vi "TLB Native Dynamic Events ver 0.08d.vi"() -> ()   [LabVIEW 2018]
uses:
  Labview Training Phase 2/Enum Controls/States for Action Engine.ctl
  Type def/TLB event states.ctl
  Type def/TLB MHL States.ctl
  <vilib>/Studica/Studica Toolkit/Background/I2C Channel.ctl
  <vilib>/myRIO/Common/Instrument Driver Framework/myRIO v1.0/AI/typedefs/AI Channels Enum.ctl
  <vilib>/myRIO/Common/Instrument Driver Framework/myRIO v1.0/AI/typedefs/AI Channels List.ctl
  Type def/Type def.ctl
  <vilib>/Studica/Studica Blackhawk/Blackhawk.lvlib
  <vilib>/Studica/Studica Toolkit/Background/Mxp Selection.ctl
  <vilib>/Studica/Studica Toolkit/Background/DIO Channel.ctl
  <vilib>/NI_Real-Time Target Support.lvlib
  <vilib>/ptbypt/NI_PtbyPt.lvlib
  <vilib>/addons/control/pid/NI_PID_pid.lvlib
  Underlying VI's/Webcam FGV Low level ver/State control.ctl
  <vilib>/userdefined/High Color/IMAQdx.ctl
  <vilib>/Studica/Studica Toolkit/NavX/NavX.lvlib
  <vilib>/addons/control/pid/pid.llb/PID (DBL).vi
  Underlying VI's/Movement control (archived)/Motor Control/States for motor control.ctl
panel:
  out "Displacement":T1
  out "Yaw":dbl
  out "Speed and distance cluster":T2
  out "Output":dbl
  in  "SENSOR":bool
  out "Decision":i8
  out "Manual Zero Yaw":bool
  in  "error in (no error)":errorcluster
  in  "RED LED State":enum16{"OFF", "ON", "BLINK"}(ring)
  in  "GREEN LED State":enum16{"OFF", "ON", "BLINK"}(ring)
  in  "Red LED":bool
  in  "Green LED":bool
  out "Input state":i8
  out "Waveform Chart 2":dbl(graph)
  out "Waveform Chart":dbl(graph)
  in  "STOP":bool
  out "DIO 0":bool
  out "DIO 1":bool
  out "Limit Switch Array":bool[](array[boolean])
  out "error out":errorcluster
  out "L/R average":fxp<+,64,64>
  out "Right Ultrasonic":fxp<+,64,16>
  out "Left Ultrasonic":fxp<+,64,16>
  out "Right IR Sensor":dbl
  out "Left IR Sensor":dbl
  out "Object detection count":T3
  out "Camera error":errorcluster
  in  "Servo Angle":u8(slide) scale=0.0..180.0
  in  "On/Off":bool
  out "Error":errorcluster
  out "element":T4
  out "Action Queue Items":i32
  out "State Logic Queue Items":i32
  out "Action Queues items":string[](array[string])=["Hardware reset", "Software reset", ""]
  out "State logic":T5=enum."Task 2"
  out "Action State":string
  # "TLB FRAMEWORK STATUS"
  # "Camera Status Loop"
  # "Test Programme written by Calvin Loke    Dated: 28 Aug 2019\nTest Programme revised by Dr Alex See   Dated 30 Aug 2019\n\nProgramme version:   TLB Native Dynamic Events ver 0.04b.vi"
  # "Problems now:\nYaw does not work when code is in last state mode\nSlow acceleration due to loop rate?"
  # "Motor Control Loop"
  # "NAVX Control Loop"
  # "Blackhawk status"
  # "Sensor data"
  # "System Health Status Update"
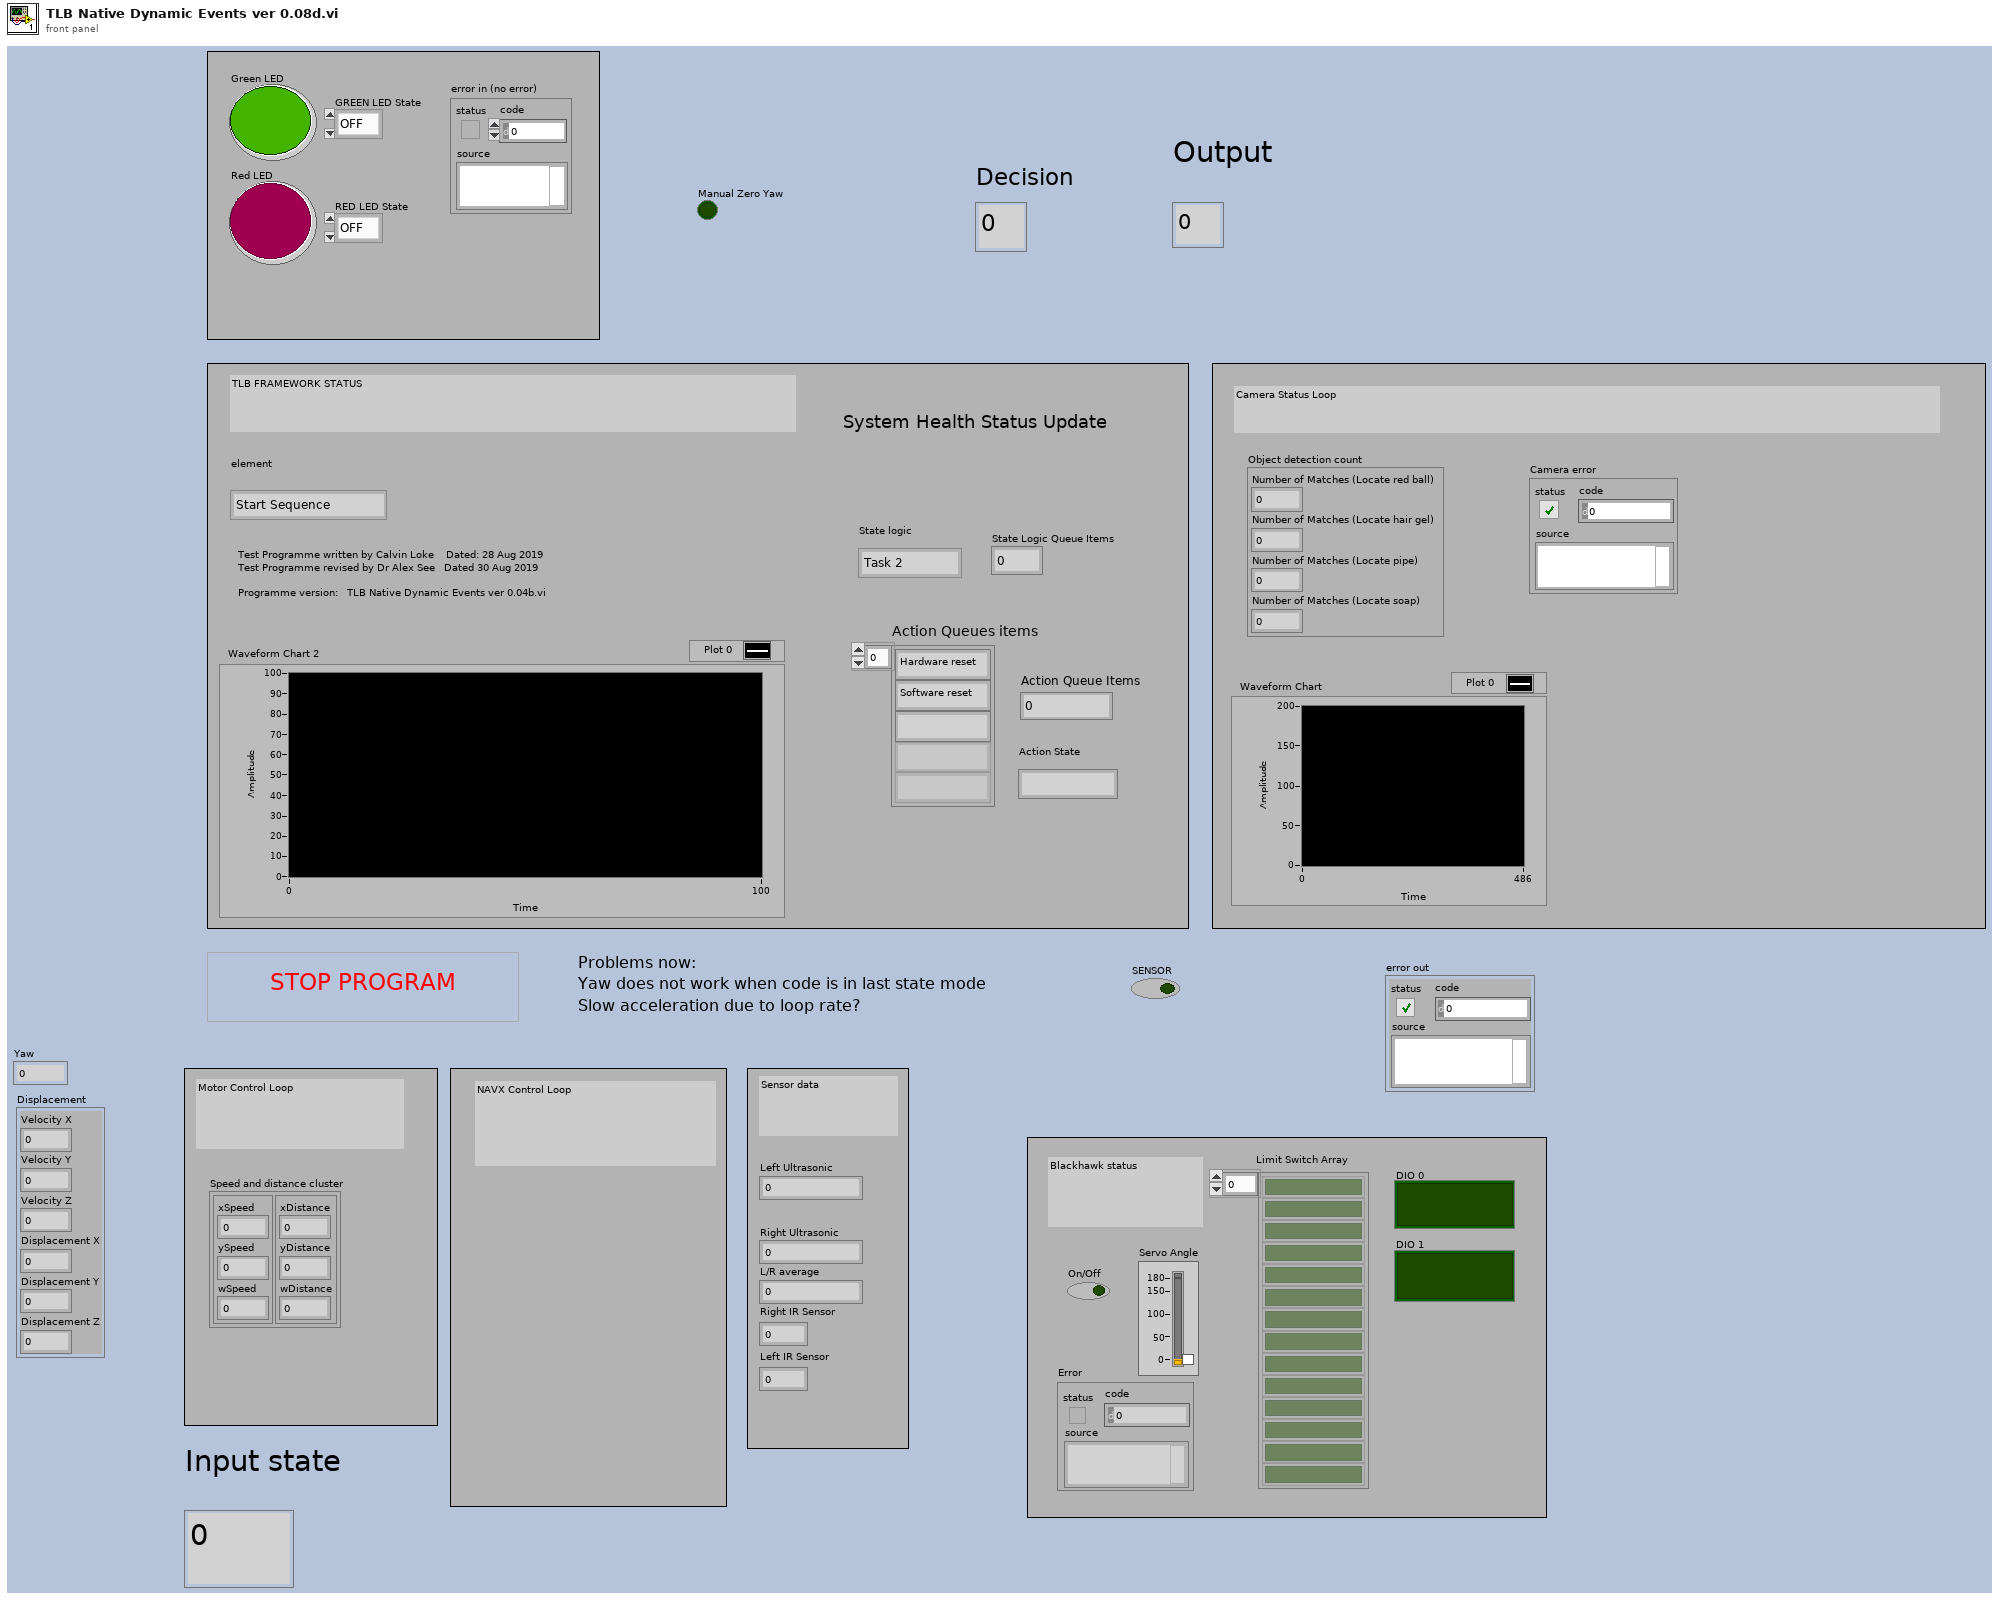
[diagram p1: front panel]
types:
  T1 = cluster{"Velocity X":dbl, "Velocity Y":dbl, "Velocity Z":dbl, "Displacement X":dbl, "Displacement Y":dbl, "Displacement Z":dbl}
  T2 = cluster{cluster{"xSpeed":dbl, "ySpeed":dbl, "wSpeed":dbl}, cluster{"xDistance":dbl, "yDistance":dbl, "wDistance":dbl}}
  T3 = cluster{"Number of Matches (Locate red ball)":i32, "Number of Matches (Locate hair gel)":i32, "Number of Matches (Locate pipe)":i32, "Number of Matches (Locate soap)":i32}
  T4 = typedef "TLB event states.ctl" = enum16{"Start Sequence", "Exit", "Start Task 1", "Start Task 2", "Start Task 3", "Start Task 4", "Camera vision", "Wall follow mode", "Idle", "Start Drive Straight"}
  T5 = typedef "TLB MHL States.ctl" = enum16{"None", "Startup", "Idle", "Processing", "Shutdown", "Reset", "Task 1", "Task 2", "Task 3", "Task 4", "Task 4a", "Task 4b", "Task 4c", "Task 4d", "Task 4e", "Task 4f", "Task 4g", "Task 4h", "Acquire image", "Wall follow mode", "Autodrive", "Autodrive a"}
  T6 = typedef "States for motor control.ctl" = enum16{"LAST STATE", "STOP", "FORWARD", "BACKWARD", "LEFT", "RIGHT", "RCW", "ACW", "INIT", "RESET ENCODERS"}
  T7 = typedef "States for Action Engine.ctl" = enum16{"Initialize", "Write", "Read"}
  T8 = typedef "DIO Channel.ctl" = enum16{"Not Connected", "A/DIO1", "A/DIO2", "A/DIO3", "A/DIO4", "A/DIO5", "A/DIO6", "A/DIO7", "A/DIO13", "B/DIO1", "B/DIO2", "B/DIO3", "B/DIO4", "B/DIO5", "B/DIO6", "B/DIO7", "B/DIO13", "C/DIO0", "C/DIO1", "C/DIO2", "C/DIO3", "C/DIO4", "C/DIO5", "C/DIO6", "C/DIO7"}
  T9 = typedef "Type def.ctl" = cluster{"Front Ultrasonic Obstruct":bool, "Left Ultrasonic Obstruct":bool, "Right Ultrasonic Obstruct ":bool}
  T10 = typedef "I2C Channel.ctl" = enum16{"Not Connected", "A", "B"}
  T11 = enum16{"LAST STATE", "STOP", "FORWARD", "BACKWARD", "LEFT", "RIGHT", "RCW", "ACW", "INIT", "RESET ENCODERS"}
  T12 = cluster{"proportional gain (Kc)":dbl, "integral time (Ti, min)":dbl, "derivative time (Td, min)":dbl}
  T13 = typedef "State control.ctl" = enum16{"Initialise", "Start camera", "Continuous Acquisition ", "Stop camera", "Dispose all"}
  T14 = typedef "IMAQdx.ctl" = refnum<k21>
  T15 = typedef "Mxp Selection.ctl" = enum16{"MXP A", "MXP B"}
  T16 = typedef "AI Channels List.ctl" = T17[]
  T17 = typedef "AI Channels Enum.ctl" = enum16{"Not Connected", "AudioIn/Left", "AudioIn/Right", "C/AI0", "C/AI1", "A/AI0", "A/AI1", "A/AI2", "A/AI3", "A/AI4", "A/AI5", "A/AI6", "A/AI7", "B/AI0", "B/AI1", "B/AI2", "B/AI3", "B/AI4", "B/AI5", "B/AI6", "B/AI7", "AI/AI0", "AI/AI1", "AI/AI2", "AI/AI3", "A/AI0 (DIFF)", "A/AI1 (DIFF)", "A/AI2 (DIFF)", "A/AI3 (DIFF)", "B/AI0 (DIFF)", "B/AI1 (DIFF)", "B/AI2 (DIFF)", "B/AI3 (DIFF)"}
  T18 = cluster{"DIO Channel":T8, "FPGA VI Reference Out":refnum<k20>}
  T19 = typedef "Analog Scaling Constants List.ctl" = T20[]
  T20 = typedef "Analog Scaling Constants.ctl" = cluster{"LSB Weight (Volts)":dbl, "Offset (Volts)":dbl, "Signed?":bool}
  T21 = cluster{"Scale Constants Array":T19, "FPGA Reference Out":refnum<k20>, "AI Channel":T16}
  T22 = cluster{"I2C Channel":T10, "FPGA VI Reference Out":refnum<k20>}
  T23 = typedef "NI_Real-Time Target Support.lvlib/RT CPU Load.ctl" = cluster{"Total (%)":dbl, "Time Critical (%)":dbl, "Timed Structures (%)":dbl, "High (%)":dbl, "Above Normal (%)":dbl, "Normal (%)":dbl, "Background (%)":dbl, "Idle (%)":dbl, "ISR (%)":dbl}
  T24 = cluster{"CPU loads[0]":T23, "CPU loads[1]":T23, "CPU loads[2]":T23, "CPU loads[3]":T23, "CPU loads[4]":T23, "CPU loads[5]":T23, "CPU loads[6]":T23, "CPU loads[7]":T23, "CPU loads[8]":T23}
  T25 = cluster{"I2C Ref Out":cluster{"I2C Channel":T10, "FPGA VI Reference Out":refnum<k20>}, "Connected":bool, "Slave Address (7-bit)":u8, "Registry":u8[]}
  T26 = typedef "IMAQ Image.ctl" = refnum<image>
  T27 = cluster{"Yaw":dbl, "Roll":dbl, "Pitch":dbl, "Heading":dbl, "Fused Heading":dbl}
  T28 = cluster{"xDistance":dbl, "yDistance":dbl, "wDistance":dbl}
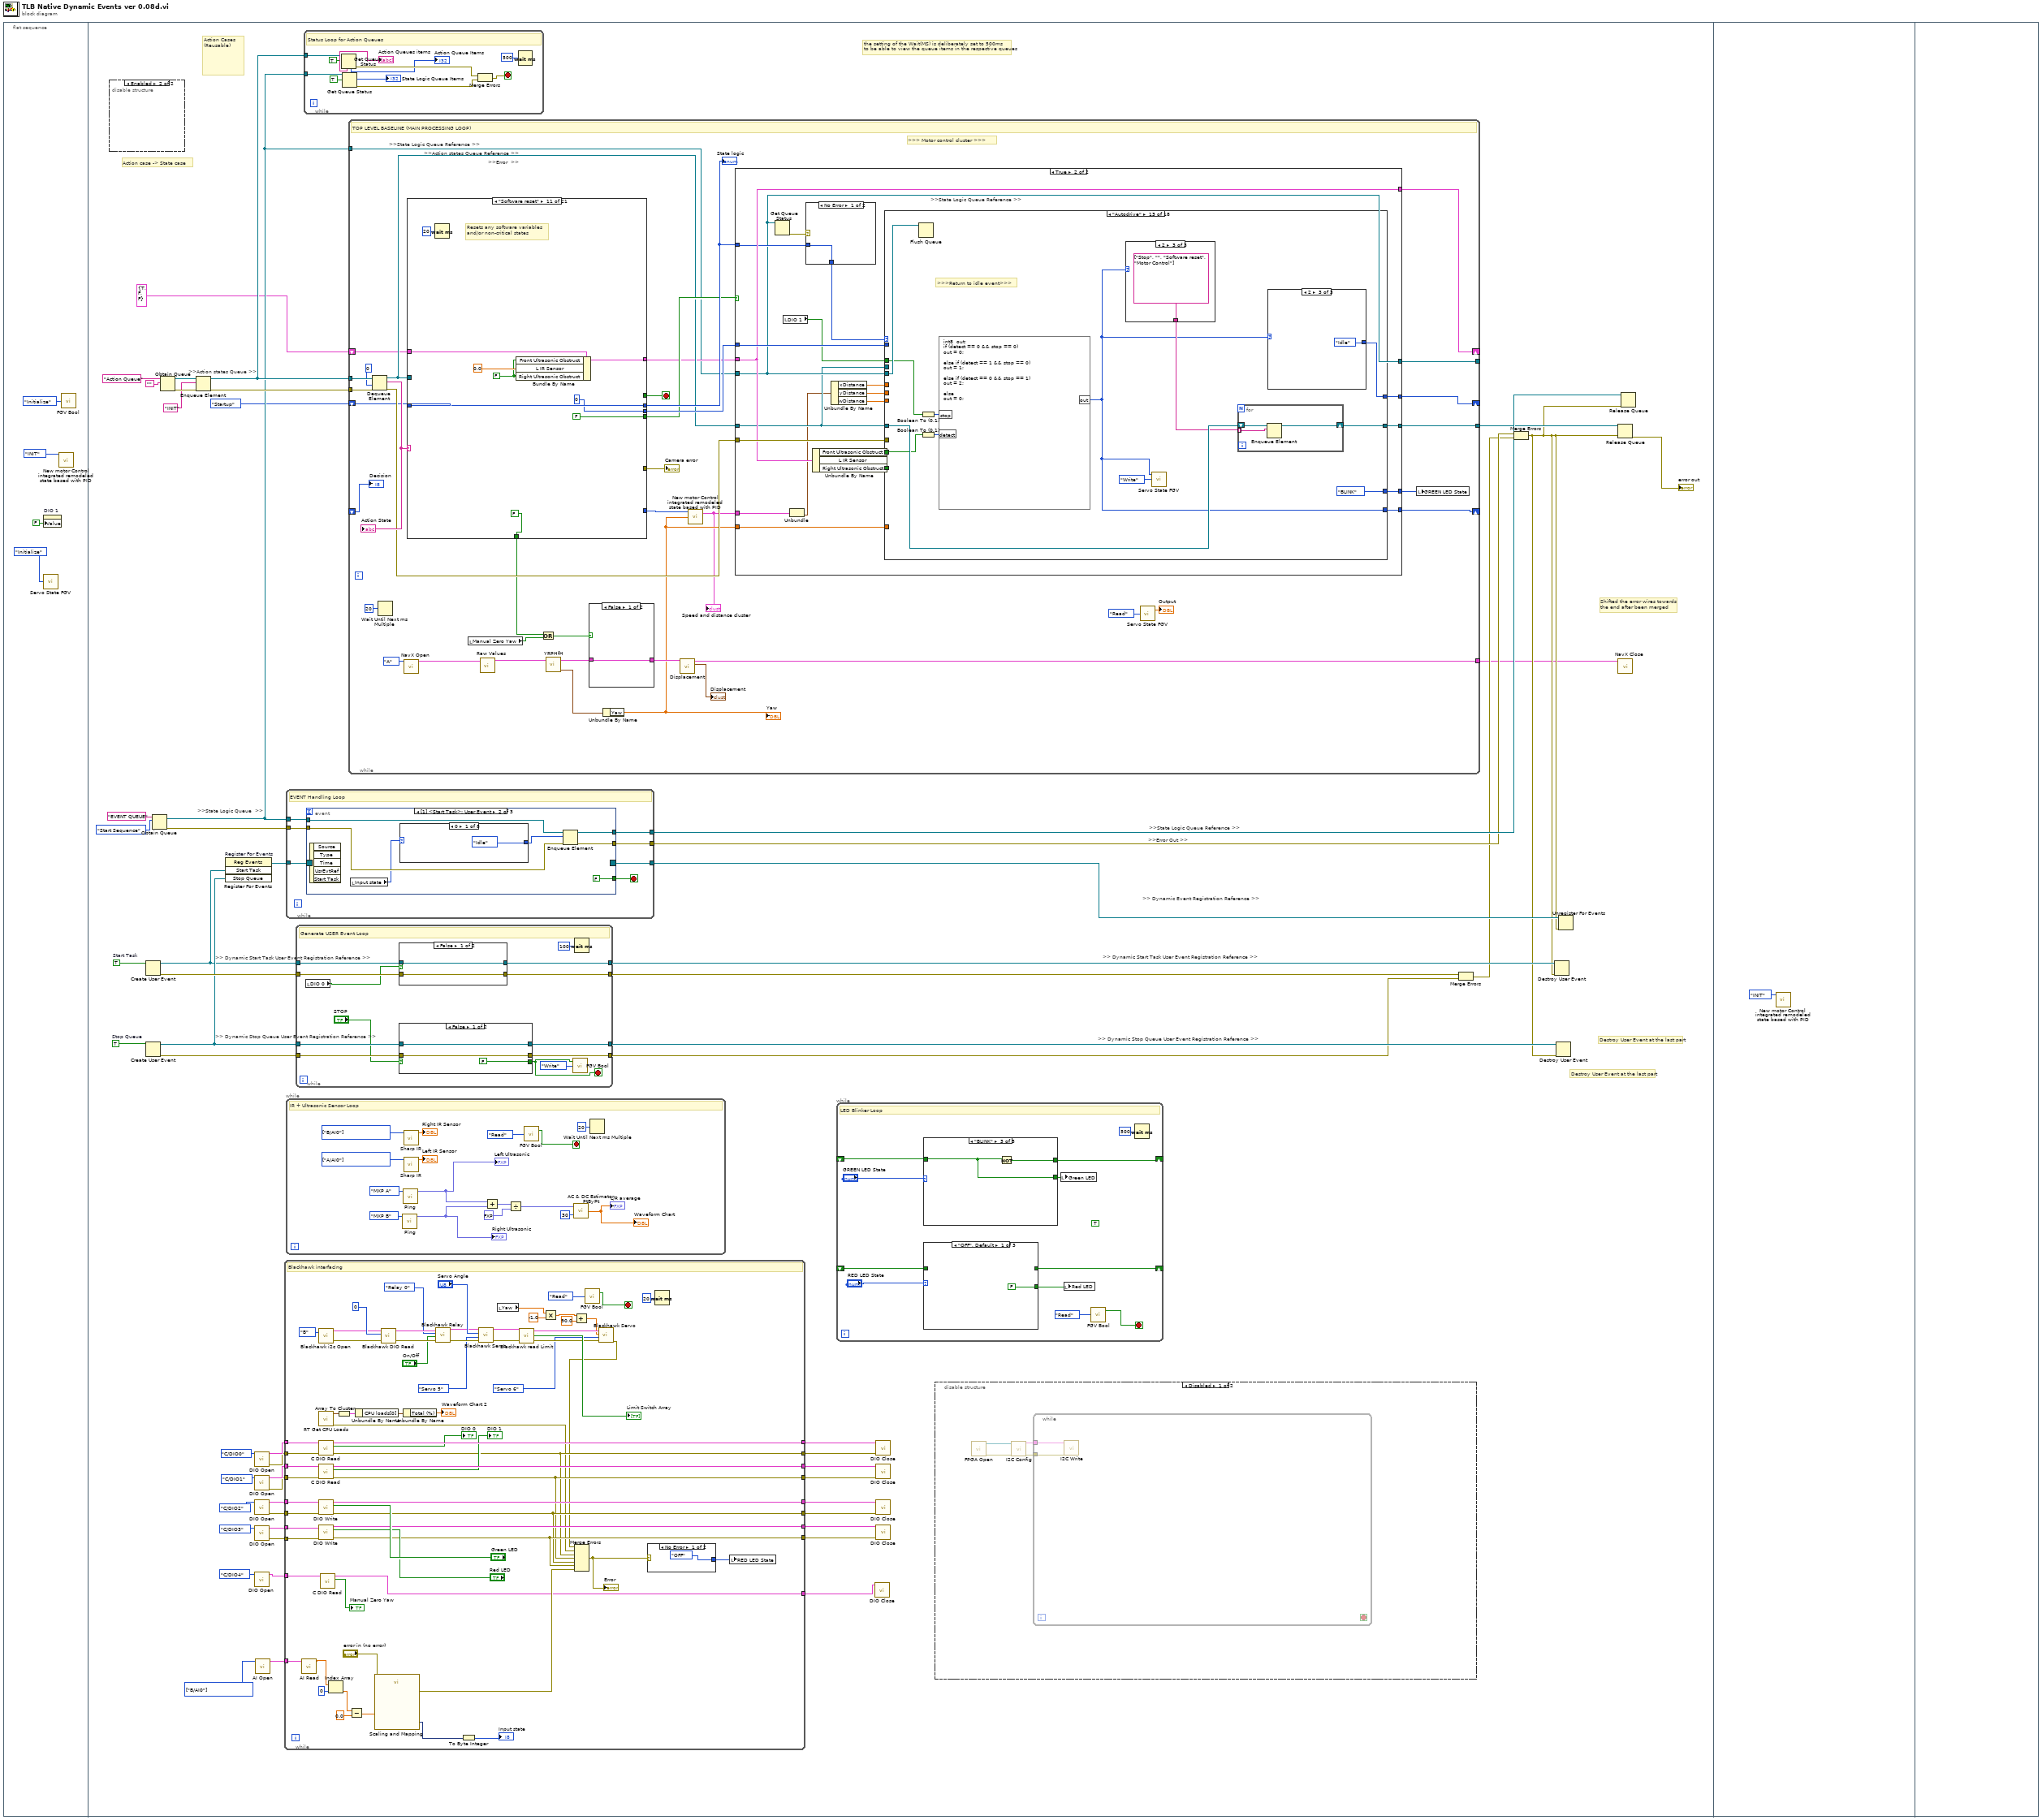
[diagram p0: block diagram]
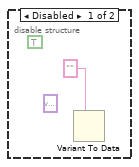
[diagram p3: hidden frame]
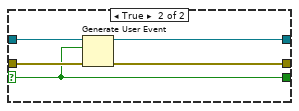
[diagram p4: hidden frame]
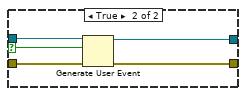
[diagram p5: hidden frame]
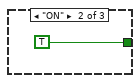
[diagram p6: hidden frame]
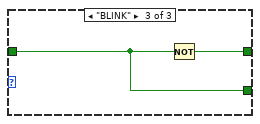
[diagram p7: hidden frame]
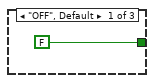
[diagram p8: hidden frame]
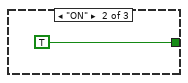
[diagram p9: hidden frame]
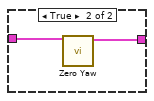
[diagram p10: hidden frame]
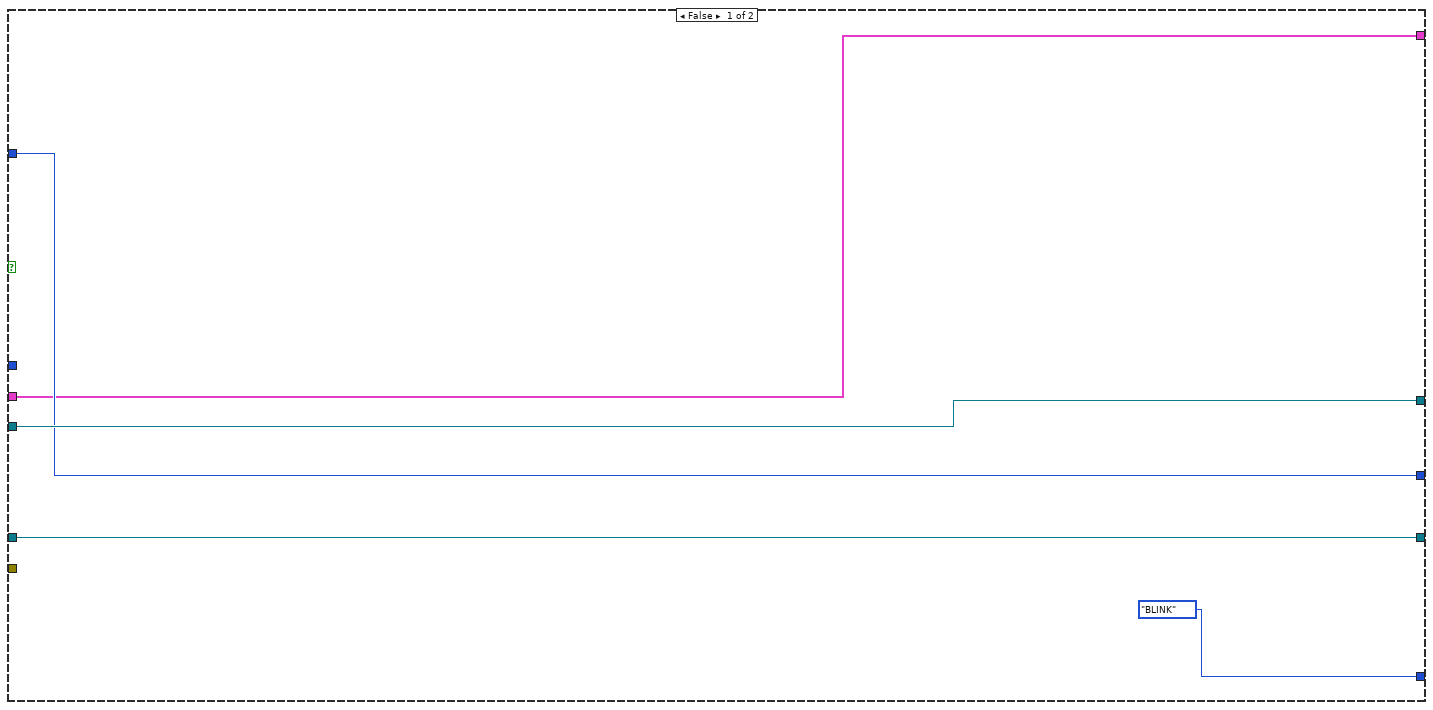
[diagram p11: hidden frame]
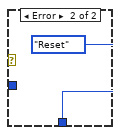
[diagram p12: hidden frame]
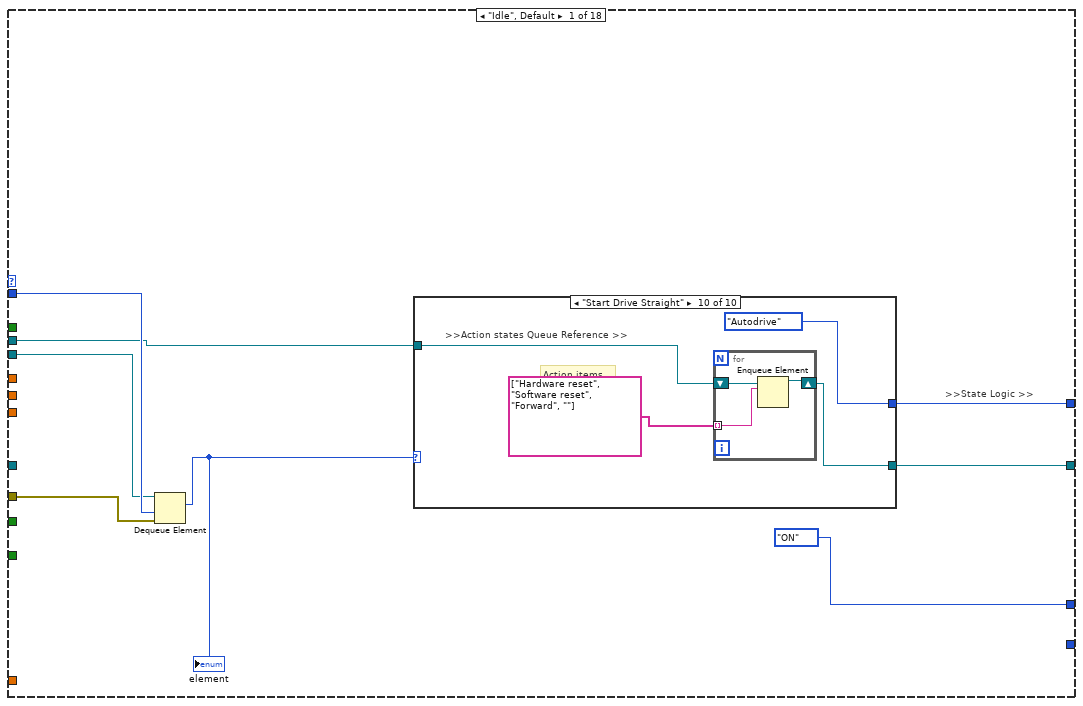
[diagram p13: hidden frame]
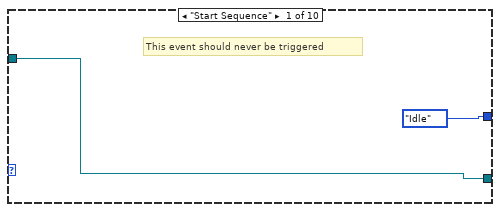
[diagram p14: hidden frame]
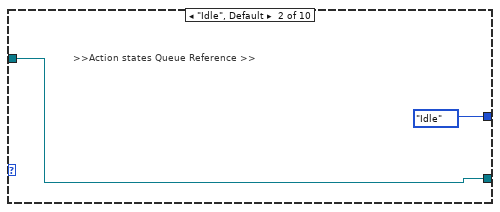
[diagram p15: hidden frame]
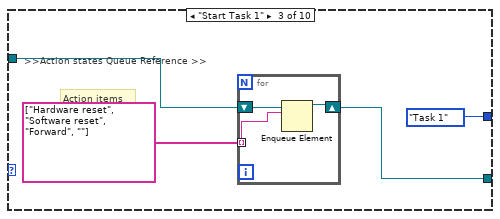
[diagram p16: hidden frame]
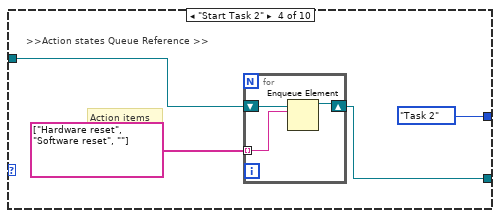
[diagram p17: hidden frame]
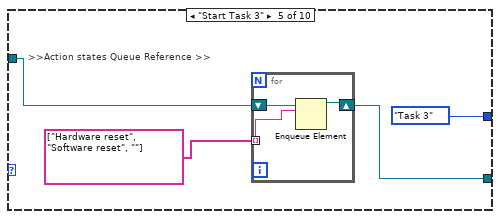
[diagram p18: hidden frame]
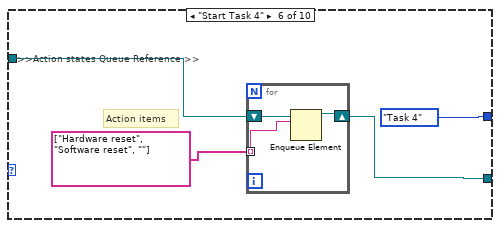
[diagram p19: hidden frame]
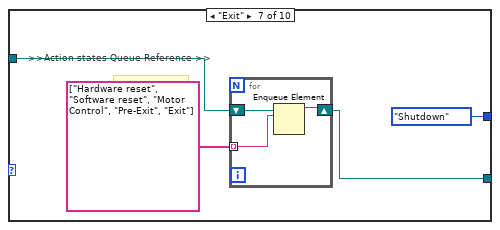
[diagram p20: hidden frame]
diagram:
  n1 = flat-sequence {
    frame #0 {
      n2 = call "Servo State FGV.vi"("Init/Read/Write State"=States_for_Action_Engine."Initialize") -> ()  [unwired: 2 in, 2 out]
      n3 = property on="DIO 1" class="Bool (strict)"("Value"=FALSE ("DIO 1")) -> ()  [unwired: 2 in, 2 out]
      n4 = call "New motor Control integrated remodeled state based with PID.vi"("States"=States_for_motor_control."INIT") -> ()  [unwired: 2 in, 2 out]
      n5 = call "FGV Bool.vi"("Init/Read/Write State"=States_for_Action_Engine."Initialize") -> ()  [unwired: 2 in, 2 out]
    }
    frame #1 {
      w14 = T16 [enum."B/AI0"] items=["Not Connected", "AudioIn/Left", "AudioIn/Right", "C/AI0", "C/AI1", "A/AI0", "A/AI1", "A/AI2", "A/AI3", "A/AI4", "A/AI5", "A/AI6", "A/AI7", "B/AI0", "B/AI1", "B/AI2", "B/AI3", "B/AI4", "B/AI5", "B/AI6", "B/AI7", "AI/AI0", "AI/AI1", "AI/AI2", "AI/AI3", "A/AI0 (DIFF)", "A/AI1 (DIFF)", "A/AI2 (DIFF)", "A/AI3 (DIFF)", "B/AI0 (DIFF)", "B/AI1 (DIFF)", "B/AI2 (DIFF)", "B/AI3 (DIFF)"] ("AI Channel")
      w61 = TRUE  # Stop Queue
      w60 = TRUE  # Start Task
      # "Action case -> State case"
      # "the setting of the Wait(MS) is deliberately set to 500ms\nto be able to view the queue items in the respective queues"
      # "Action Cases\n(Reusable)"
      # ">>Error Out >>"
      # ">> Dynamic Stop Queue User Event Registration Reference >>"
      # ">> Dynamic Start Task User Event Registration Reference >>"
      # ">> Dynamic Stop Queue User Event Registration Reference >>"
      # ">> Dynamic Start Task User Event Registration Reference >>"
      # ">> Dynamic Event Registration Reference >>"
      # ">>Action states Queue >>"
      # ">>State Logic Queue  >>"
      # ">>State Logic Queue Reference >>"
      # "Destroy User Event at the last part"
      # "Destroy User Event at the last part"
      # "Shifted the error wires towards\nthe end after been merged"
      n6 = disable-structure shown="Enabled" {
        frame Disabled {
          (unwired) variant
          (unwired) TRUE
          n7 = Variant To Data(type="") -> ()  [unwired: 2 in, 2 out]
        }
        frame Enabled {
        }
      }
      n8 = Create User Event(user event datatype=w60) -> (user event=w52:refnum<user-event>, error out=w57:errorcluster)  [unwired: 1 in]
      n9 = Create User Event(user event datatype=w61) -> (user event=w53:refnum<user-event>, error out=w56:errorcluster)  [unwired: 1 in]
      n10 = Obtain Queue(name (unnamed)="EVENT QUEUE", element data type=TLB_event_states."Start Sequence" ("Enum")) -> (queue out=w37:refnum<queue>, error out=w43:errorcluster)  [unwired: 3 in, 1 out]
      n11 = Obtain Queue(name (unnamed)="Action Queue", element data type="") -> (queue out=w46:refnum<queue>, error out=w42:errorcluster)  [unwired: 3 in, 1 out]
      n12 = Enqueue Element(queue=w46, element="INIT", error in (no error)=w42) -> (queue out=w38:refnum<queue>, error out=w41:errorcluster)  [unwired: 1 in, 1 out]
      n13 = register-events "Register For Events"(w52, w53) -> (reference out=w51:refnum<event-registration>)  [unwired: 2 in, 1 out]
      n14 = call <vilib>:"DIO Open.vi"("DIO Channel"=DIO_Channel."C/DIO4") -> ("DIO Info Out"=w8:T18)  [unwired: 9 in, 1 out]
      n15 = call <vilib>:"DIO Open.vi"("DIO Channel"=DIO_Channel."C/DIO0") -> ("error out"=w24:errorcluster, "DIO Info Out"=w30:T18)  [unwired: 9 in]
      n16 = call <vilib>:"DIO Open.vi"("DIO Channel"=DIO_Channel."C/DIO1") -> ("error out"=w22:errorcluster, "DIO Info Out"=w26:T18)  [unwired: 9 in]
      n17 = call <vilib>:"DIO Open.vi"("DIO Channel"=DIO_Channel."C/DIO2") -> ("error out"=w12:errorcluster, "DIO Info Out"=w18:T18)  [unwired: 9 in]
      n18 = call <vilib>:"DIO Open.vi"("DIO Channel"=DIO_Channel."C/DIO3") -> ("error out"=w10:errorcluster, "DIO Info Out"=w17:T18)  [unwired: 9 in]
      n19 = call <vilib>:"AI Open.vi"("AI Channel"=w14) -> ("Analog Info"=w13:T21)  [unwired: 9 in, 1 out]
      n20 = while {
        tunnel: w30 -> [w743]
        tunnel: [w742] -> w29
        tunnel: w26 -> [w741]
        tunnel: [w740] -> w25
        tunnel: w24 -> [w739]
        tunnel: [w708] -> w23
        tunnel: w22 -> [w738]
        tunnel: [w709] -> w21
        tunnel: w18 -> [w732]
        tunnel: w17 -> [w731]
        tunnel: [w728] -> w16
        tunnel: [w727] -> w15
        tunnel: w13 -> [w726]
        tunnel: w12 -> [w719]
        tunnel: [w710] -> w11
        tunnel: w10 -> [w718]
        tunnel: [w711] -> w9
        tunnel: w8 -> [w699]
        tunnel: [w698] -> w6
        stop <- w756 stop-if-true
        # "Blackhawk interfacing"
        n21 = call <vilib>:"AI Read.vi"("Analog Info"=w726) -> ("Array"=w722:dbl[])  [unwired: 9 in, 1 out]
        n22 = call <vilib>:"Blackhawk i2c Open.vi"("I2C Channel"=I2C_Channel."B") -> ("I2C Ref Out"=w734:T22, "error out"=w733:errorcluster)  [unwired: 2 in]
        n23 = call <vilib>:"RT Get CPU Loads.vi"() -> ("error out"=w707:errorcluster, "CPU loads"=w713:T23[])  [unwired: 10 in]
        n24 = call <vilib>:"C DIO Read.vi"("error in (no error)"=w739, "DIO Info In in"=w743) -> ("error out"=w708:errorcluster, "IN"=→"DIO 0":bool, "DIO Info In out"=w742:T18)  [unwired: 7 in]
        n25 = call <vilib>:"C DIO Read.vi"("error in (no error)"=w738, "DIO Info In in"=w741) -> ("error out"=w709:errorcluster, "IN"=→"DIO 1":bool, "DIO Info In out"=w740:T18)  [unwired: 7 in]
        n26 = call <vilib>:"DIO Write.vi"("error in (no error)"=w719, "Input"="Green LED", "DIO Info In"=w732) -> ("error out"=w710:errorcluster, "DIO Info Out"=w728:T18)  [unwired: 7 in]
        n27 = call <vilib>:"DIO Write.vi"("error in (no error)"=w718, "Input"="Red LED", "DIO Info In"=w731) -> ("error out"=w711:errorcluster, "DIO Info Out"=w727:T18)  [unwired: 7 in]
        n28 = call <vilib>:"C DIO Read.vi"("DIO Info In in"=w699) -> ("IN"=→"Manual Zero Yaw":bool, "DIO Info In out"=w698:T18)  [unwired: 8 in, 1 out]
        n29 = Index Array(array=w722, index=0) -> (element=w724:dbl)
        n30 = Array To Cluster(array=w713) -> (cluster=w714:T24)
        n31 = Subtract(x=w724, y=0.0) -> (x-y=w725:dbl)
        n32 = Unbundle By Name(w714) -> ("CPU loads[0]"=w715:T23)
        n33 = call "Scaling and Mapping"("error in (no error)"="error in (no error)", "Signals"=w725) -> ("error out"=w712:errorcluster, "Scaled Signals"=w720:dynamicdata)  [unwired: 8 in]
        n34 = call <vilib>:"Blackhawk DIO Read.vi"("I2C Ref In"=w734, "PIN"=u8 0, "error in (no error)"=w733) -> ("I2C Ref Out"=w754:T22, "error out"=w755:errorcluster)  [unwired: 3 in, 1 out]
        n35 = Unbundle By Name(w715) -> ("Total (%)"=→"Waveform Chart 2":dbl)
        n36 = call <vilib>:"Blackhawk Relay.vi"("error in (no error)"=w755, "On/Off"="On/Off", "Relay"=enum8{"Relay 0", "Relay 1", "Relay 2"}."Relay 0", "I2C Ref In"=w754) -> ("error out"=w751:errorcluster, "I2C Ref Out"=w748:T22)  [unwired: 6 in]
        n37 = To Byte Integer(number=w720) -> (8bit integer=→"Input state":i8)
        n38 = call <vilib>:"Blackhawk Servo.vi"("error in (no error)"=w751, "Servo Select"=enum16{"Servo 5", "Servo 6"}."Servo 5", "Servo Angle"="Servo Angle", "I2C Ref In"=w748) -> ("error out"=w746:errorcluster, "I2C Ref Out"=w745:T22)  [unwired: 6 in]
        n39 = local read "Yaw"() -> (w692:dbl)
        n40 = call <vilib>:"Blackhawk read Limit.vi"("error in (no error)"=w746, "I2C Ref In"=w745) -> ("error out"=w703:errorcluster, "Limit Switch Array"=→"Limit Switch Array":bool[], "I2C Ref Out"=w701:T22)  [unwired: 1 in]
        n41 = Multiply(x=w692, y=-1.0) -> (x*y=w694:dbl)
        n42 = Add(x=w694, y=90.0) -> (x+y=w695:dbl)
        n43 = call "FGV Bool.vi"("Init/Read/Write State"=States_for_Action_Engine."Read") -> ("Output node"=w756:bool)  [unwired: 2 in, 1 out]
        n44 = call <vilib>:"Blackhawk Servo.vi"("error in (no error)"=w703, "Servo Select"=enum16{"Servo 5", "Servo 6"}."Servo 6", "Servo Angle"=w695, "I2C Ref In"=w701) -> ("error out"=w702:errorcluster)  [unwired: 6 in, 1 out]
        n45 = Merge Errors(w702, w707, w708, w709, w710, w711, w712) -> (w706:errorcluster)
        "Error" <- w706
        n46 = case shown="No Error" w706 {
          tunnel: [enum16{"OFF", "ON", "BLINK"}."OFF" ("RED LED State") enum16{"OFF", "ON", "BLINK"}."BLINK" ("RED LED State")] -> w717
          frame No Error {
          }
          frame Error {
          }
        }
        n47 = Wait (ms)(milliseconds to wait=u32 20) -> ()  [unwired: 1 out]
        n48 = local write "RED LED State"(w717) -> ()
      }
      n49 = while {
        tunnel: w51 -> [w664]
        tunnel: [w663] -> w50
        tunnel: w37 -> [w661]
        tunnel: [w660] -> w49
        tunnel: w43 -> [w659]
        tunnel: [w658] -> w40
        stop <- w662 stop-if-true
        # "EVENT Handling Loop"
        n50 = event shown="[1] <Start Task>: User Event" {
          selector: w664 -> [_ _ _]
          dyn-events: [_ _ _] -> w663
          timeout: _ -> [_ _ _]
          tunnel: [FALSE FALSE w691] -> w662
          tunnel: w661 -> [w669 w676 w689]
          tunnel: [w668 w675 w690] -> w660
          tunnel: w659 -> [w666 w674 w687]
          tunnel: [w665 w673 w686] -> w658
          event Timeout {
            n51 = event-data() -> ()  [unwired: 1 in, 3 out]
            n52 = Enqueue Element(queue=w669, element=TLB_event_states."Idle" ("Enum"), error in (no error)=w666) -> (queue out=w668:refnum<queue>, error out=w665:errorcluster)  [unwired: 1 in, 1 out]
          }
          event User Event {
            n53 = event-data() -> ()  [unwired: 1 in, 5 out]
            n54 = local read "Input state"() -> (w672:i8)
            n55 = case shown="0" w672 {
              tunnel: [TLB_event_states."Idle" ("Enum") TLB_event_states."Start Task 1" ("Enum") TLB_event_states."Start Task 2" ("Enum") TLB_event_states."Start Task 3" ("Enum") TLB_event_states."Start Task 4" ("Enum") TLB_event_states."Wall follow mode" ("Enum") TLB_event_states."Camera vision" ("Enum") TLB_event_states."Start Drive Straight" ("Enum")] -> w671
              frame 0 {
              }
              frame 1 {
              }
              frame 2 {
              }
              frame 3, Default {
              }
              frame 4 {
              }
              frame 5 {
              }
              frame 6 {
              }
              frame 7 {
              }
            }
            n56 = Enqueue Element(queue=w676, element=w671, error in (no error)=w674) -> (queue out=w675:refnum<queue>, error out=w673:errorcluster)  [unwired: 1 in, 1 out]
          }
          event User Event {
            n57 = event-data() -> ("Stop Queue"=w691:bool)  [unwired: 1 in, 4 out]
            n58 = Enqueue Element At Opposite End(queue=w689, element=TLB_event_states."Exit" ("Enum"), error in (no error)=w687) -> (queue out=w690:refnum<queue>, error out=w686:errorcluster)  [unwired: 1 in, 1 out]
          }
        }
      }
      n59 = while {
        stop <- w651 stop-if-true
        w656 = T16 [enum."A/AI0"] items=["Not Connected", "AudioIn/Left", "AudioIn/Right", "C/AI0", "C/AI1", "A/AI0", "A/AI1", "A/AI2", "A/AI3", "A/AI4", "A/AI5", "A/AI6", "A/AI7", "B/AI0", "B/AI1", "B/AI2", "B/AI3", "B/AI4", "B/AI5", "B/AI6", "B/AI7", "AI/AI0", "AI/AI1", "AI/AI2", "AI/AI3", "A/AI0 (DIFF)", "A/AI1 (DIFF)", "A/AI2 (DIFF)", "A/AI3 (DIFF)", "B/AI0 (DIFF)", "B/AI1 (DIFF)", "B/AI2 (DIFF)", "B/AI3 (DIFF)"] ("AI Channel")
        w657 = T16 [enum."B/AI0"] items=["Not Connected", "AudioIn/Left", "AudioIn/Right", "C/AI0", "C/AI1", "A/AI0", "A/AI1", "A/AI2", "A/AI3", "A/AI4", "A/AI5", "A/AI6", "A/AI7", "B/AI0", "B/AI1", "B/AI2", "B/AI3", "B/AI4", "B/AI5", "B/AI6", "B/AI7", "AI/AI0", "AI/AI1", "AI/AI2", "AI/AI3", "A/AI0 (DIFF)", "A/AI1 (DIFF)", "A/AI2 (DIFF)", "A/AI3 (DIFF)", "B/AI0 (DIFF)", "B/AI1 (DIFF)", "B/AI2 (DIFF)", "B/AI3 (DIFF)"] ("AI Channel")
        # "IR + Ultrasonic Sensor Loop"
        n60 = call <vilib>:"Ping.vi"("Mxp Side"=Mxp_Selection."MXP B") -> ("CM"=w645:fxp<+,64,16>)  [unwired: 8 in, 2 out]
        "Right Ultrasonic" <- w645
        n61 = call <vilib>:"Ping.vi"("Mxp Side"=Mxp_Selection."MXP A") -> ("CM"=w646:fxp<+,64,16>)  [unwired: 8 in, 2 out]
        "Left Ultrasonic" <- w646
        n62 = call <vilib>:"Sharp IR.vi"("AI Channel"=w657) -> ("Sharp IR Distance"=→"Right IR Sensor":dbl)  [unwired: 8 in, 2 out]
        n63 = call <vilib>:"Sharp IR.vi"("AI Channel"=w656) -> ("Sharp IR Distance"=→"Left IR Sensor":dbl)  [unwired: 8 in, 2 out]
        n64 = Add(x=w646, y=w645) -> (x+y=w648:fxp<+,64,17>)
        n65 = Divide(x=w648, y=fxp<+,64,17> 2.0) -> (x/y=w644:fxp<+,64,64>)
        n66 = call "FGV Bool.vi"("Init/Read/Write State"=States_for_Action_Engine."Read") -> ("Output node"=w651:bool)  [unwired: 2 in, 1 out]
        n67 = call <vilib>:"AC & DC Estimator PtByPt.vi"("signal"=w644, "sample length"=30) -> ("DC estimate (V)"=→"L/R average" →"Waveform Chart":dbl)  [unwired: 1 in, 2 out]
        n68 = Wait Until Next ms Multiple(millisecond multiple=u32 20) -> ()  [unwired: 1 out]
      }
      n69 = while {
        tunnel: w52 -> [w91]
        tunnel: w53 -> [w90]
        tunnel: [w89] -> w59
        tunnel: [w88] -> w58
        tunnel: w57 -> [w87]
        tunnel: [w86] -> w55
        tunnel: w56 -> [w85]
        tunnel: [w84] -> w54
        stop <- w82 stop-if-true
        # "Generate USER Event Loop"
        n70 = local read "DIO 0"() -> (w81:bool)
        n71 = case shown="False" w81 {
          selector: w81 -> [_ w103]
          tunnel: w91 -> [w102 w107]
          tunnel: [w102 w106] -> w88
          tunnel: w87 -> [w101 w105]
          tunnel: [w101 w104] -> w86
          frame False {
          }
          frame True {
            n72 = Generate User Event(user event=w107, event data cluster=w103, error in=w105) -> (user event out=w106:refnum<user-event>, error out=w104:errorcluster)  [unwired: 1 in]
          }
        }
        n73 = case shown="False" "STOP" {
          selector: "STOP" -> [_ w96]
          tunnel: w90 -> [w95 w100]
          tunnel: [w95 w99] -> w89
          tunnel: w85 -> [w94 w98]
          tunnel: [w94 w97] -> w84
          tunnel: [FALSE w96] -> w82
          frame False {
          }
          frame True {
            n74 = Generate User Event(user event=w100, event data cluster=w96, error in=w98) -> (user event out=w99:refnum<user-event>, error out=w97:errorcluster)  [unwired: 1 in]
          }
        }
        n75 = call "FGV Bool.vi"("Init/Read/Write State"=States_for_Action_Engine."Write", "Input Node"=w82) -> ()  [unwired: 1 in, 2 out]
        n76 = Wait (ms)(milliseconds to wait=u32 100) -> ()  [unwired: 1 out]
      }
      n77 = while {
        tunnel: w38 -> [w77]
        tunnel: w37 -> [w74]
        stop <- w71 stop-if-true
        # "Status Loop for Action Queues"
        n78 = Get Queue Status(queue=w77, return elements? (F)=TRUE) -> (error out=w73:errorcluster, # elements in queue=→"Action Queue Items":i32, elements=→"Action Queues items":string[])  [unwired: 1 in, 5 out]
        n79 = Get Queue Status(queue=w74, return elements? (F)=TRUE) -> (# pending remove=→"State Logic Queue Items":i32, error out=w72:errorcluster)  [unwired: 1 in, 6 out]
        n80 = Merge Errors(w73, w72) -> (w71:errorcluster)
        n81 = Wait (ms)(milliseconds to wait=u32 500) -> ()  [unwired: 1 out]
      }
      n82 = while {
        tunnel: w37 -> [w148]
        shift-right: [w159] -> _
        shift-left: TLB_MHL_States."Startup" ("Enum") -> [w153]
        tunnel: w38 -> [w164]
        tunnel: w41 -> [w162]
        tunnel: [w161] -> _
        tunnel: [w160] -> w33
        shift-right: [w150] -> _
        shift-left: T9 {"Front Ultrasonic Obstruct"=TRUE, "Left Ultrasonic Obstruct"=FALSE, "Right Ultrasonic Obstruct "=FALSE} -> [w152]
        shift-right: [w144] -> _
        shift-left: _ -> [w143]
        tunnel: [w133] -> w5
        stop <- w146 stop-if-true
        # ">>> Motor control cluster >>>"
        # ">>Error  >>"
        # ">>Action states Queue Reference >>"
        # ">>State Logic Queue Reference >>"
        # "TOP LEVEL BASELINE (MAIN PROCESSING LOOP)"
        n83 = Dequeue Element(queue=w164, timeout in ms (-1)=0, error in (no error)=w162) -> (queue out=w154:refnum<queue>, element=w163:string, error out=w155:errorcluster)  [unwired: 1 out]
        "Action State" <- w163
        n84 = Wait Until Next ms Multiple(millisecond multiple=u32 20) -> ()  [unwired: 1 out]
        n85 = call <vilib>:"NavX Open.vi"("I2C Channel"=I2C_Channel."A") -> ("NavX Info"=w136:T25)  [unwired: 9 in, 1 out]
        n86 = case shown="\"Software reset\"" w163 {
          tunnel: [w496 w511 w517 w522 w527 w533 w538 w541 w548 w553 w563 w570 TLB_MHL_States."Shutdown" ("Enum") w580 w591 w594 w605 w616 w624 w636 w640] -> w165
          tunnel: [w499 0 0 0 0 0 0 0 0 0 0 0 0 0 0 0 0 0 0 0 0] -> w158
          tunnel: [TRUE FALSE FALSE FALSE FALSE FALSE FALSE FALSE FALSE FALSE FALSE FALSE FALSE FALSE FALSE FALSE FALSE FALSE FALSE FALSE FALSE] -> w157
          tunnel: w154 -> [_ _ _ _ _ _ _ _ _ _ _ _ _ _ _ _ _ _ _ _ _]
          tunnel: w153 -> [w496 w511 w517 w522 w527 w533 w538 w541 w548 w553 w563 w570 _ w580 w591 w594 w605 w616 w624 w636 w640]
          tunnel: w152 -> [w497 w506 w514 w523 w525 w530 w535 w540 w545 w551 w560 w567 w573 w581 w590 w597 w606 w617 w623 w633 w641]
          tunnel: [w497 w505 w513 w523 w525 w530 w535 w540 w545 w551 w559 w567 w573 w581 w587 w596 w606 w617 w623 w633 w641] -> w151
          tunnel: [_ _ _ _ _ _ _ _ _ _ _ _ _ _ _ _ _ w607 w619 w627 _] -> w149
          tunnel: [_ _ _ _ _ _ _ _ _ _ _ _ TRUE _ _ _ _ _ _ _ _] -> w146
          tunnel: [T11."LAST STATE" ("Move mode") T11."INIT" ("Move mode") T11."FORWARD" ("Move mode") T11."LAST STATE" ("Move mode") T11."BACKWARD" ("Move mode") T11."RIGHT" ("Move mode") T11."LEFT" ("Move mode") T11."RCW" ("Move mode") T11."ACW" ("Move mode") T11."STOP" ("Move mode") _ T11."RESET ENCODERS" ("Move mode") T11."INIT" ("Move mode") T11."INIT" ("Move mode") _ _ _ _ _ _ _] -> w129
          tunnel: [FALSE ("NavX Zero Yaw") _ _ _ _ _ _ _ _ FALSE ("NavX Zero Yaw") FALSE ("NavX Zero Yaw") TRUE ("NavX Zero Yaw") _ _ _ _ _ _ _ _ _] -> w130
          frame "No action", Default {
            n87 = case shown="\"Startup\", Default" w496 {
              tunnel: [0 100] -> w499
              frame "Startup", Default {
              }
              frame "Idle" {
              }
            }
          }
          frame "Init" {
            # ">>State Logic  >>"
            n88 = local write "Servo Angle"(u8 90 ("Servo Angle")) -> ()
            n89 = Bundle By Name(cluster=w506, "Front Ultrasonic Obstruct"=FALSE ("Object detected"), "L IR Sensor"=0.0, "Right Ultrasonic Obstruct"=FALSE ("In move state?")) -> (w505:T9)
          }
          frame "Forward" {
            n90 = Bundle By Name(cluster=w514, "Right Ultrasonic Obstruct"=TRUE ("In move state?")) -> (w513:T9)
          }
          frame " Motor Control" {
          }
          frame "Reverse" {
          }
          frame "Right" {
          }
          frame "Left" {
          }
          frame "Rotate CW" {
          }
          frame "Rotate ACW" {
          }
          frame "Stop" {
          }
          frame "Software reset" {
            w555 = FALSE ("In move state?")
            # "Resets any software variables\nand/or non-critical states"
            n91 = Wait (ms)(milliseconds to wait=u32 20) -> ()  [unwired: 1 out]
            n92 = Bundle By Name(cluster=w560, "Front Ultrasonic Obstruct"=w555, "L IR Sensor"=0.0, "Right Ultrasonic Obstruct"=w555) -> (w559:T9)
          }
          frame "Hardware reset" {
            n93 = Wait (ms)(milliseconds to wait=u32 100) -> ()  [unwired: 1 out]
          }
          frame "Exit" {
          }
          frame "Pre-Exit" {
          }
          frame "Ultrasonic read" {
            # "Object detection"
            n94 = local read "L/R average"() -> (w585:fxp<+,64,64>)
            n95 = Less Or Equal?(x=w585, y=35.0) -> (x <= y?=w584:bool)
            n96 = Or(x=w584, y="SENSOR") -> (x .or. y?=w583:bool)
            n97 = Bundle By Name(cluster=w590, "Front Ultrasonic Obstruct"=w583) -> (w587:T9)
          }
          frame "IR Sensor Read" {
            n98 = local read "Left IR Sensor"() -> (w595:dbl)
            n99 = Bundle By Name(cluster=w597, "L IR Sensor"=w595) -> (w596:T9)
          }
          frame "Calculate" {
            n100 = Unbundle By Name(w606) -> ("L IR Sensor"=w601:dbl)
            n101 = call-poly <vilib>:"PID.vi"("output range"=cluster{"output high":dbl, "output low":dbl} {"output high"=0.3, "output low"=-0.3}, "PID gains"=T12 {"proportional gain (Kc)"=0.01, "integral time (Ti, min)"=0.0, "derivative time (Td, min)"=0.0}, "process variable"=w601, "setpoint"=20.0) -> ("output"=w598:dbl)  [unwired: 6 in, 1 out]
            n102 = Negate(x=w598) -> ()  [unwired: 1 out]
          }
          frame "Cam Init" {
            n103 = call "Low-Level Grab.vi"("States"=State_control."Initialise", "Session In"=T14 "cam1") -> ("error out"=w608:errorcluster, "Session Out"=w609:T14)  [unwired: 7 in, 1 out]
            n104 = call "Low-Level Grab.vi"("error in (no error)"=w608, "States"=State_control."Start camera", "Session In"=w609) -> ("error out"=w607:errorcluster)  [unwired: 6 in, 2 out]
            n105 = local write "Servo Angle"(u8 170 ("Servo Angle")) -> ()
          }
          frame "Cam Acq" {
            n106 = call "Low-Level Grab.vi"("States"=State_control."Continuous Acquisition ") -> ("error out"=w620:errorcluster, "Image Out"=w621:T26)  [unwired: 8 in, 1 out]
            n107 = call "All object detection ver2.vi"("Image In"=w621, "error in"=w620) -> ("Object detection count"=→"Object detection count":T3, "error out"=w619:errorcluster)  [unwired: 1 out]
          }
          frame "Cam Exit" {
            n108 = call "Low-Level Grab.vi"("States"=State_control."Stop camera") -> ("error out"=w628:errorcluster, "Session Out"=w630:T14)  [unwired: 8 in, 1 out]
            n109 = local write "Servo Angle"(u8 90 ("Servo Angle")) -> ()
            n110 = call "Low-Level Grab.vi"("error in (no error)"=w628, "States"=State_control."Dispose all", "Session In"=w630) -> ("error out"=w627:errorcluster)  [unwired: 6 in, 2 out]
          }
          frame "NavX Calibrate" {
            # "Adds a 15 second delay to the startup process \nfor the NavX to calibrate"
            n111 = Wait (ms)(milliseconds to wait=u32 15000) -> ()  [unwired: 1 out]
          }
        }
        "State logic" <- w165
        "Camera error" <- w149
        n112 = local read "Manual Zero Yaw"() -> (w131:bool)
        n113 = call <vilib>:"Raw Values.vi"("NavX Info In"=w136) -> ("NavX Info Out"=w139:T25)  [unwired: 8 in, 1 out]
        n114 = Or(x=w130, y=w131) -> (x .or. y?=w132:bool)
        n115 = call <vilib>:"YRPHfH.vi"("NavX Info In"=w139) -> ("YRPHfH"=w140:T27, "NavX Info Out"=w138:T25)  [unwired: 3 in]
        n116 = case shown="False" w132 {
          tunnel: [w166 w168] -> w135
          tunnel: w138 -> [w166 w167]
          frame False {
          }
          frame True {
            n117 = call <vilib>:"Zero Yaw.vi"("NavX Info In"=w167) -> ("NavX Info Out"=w168:T25)  [unwired: 10 in]
          }
        }
        n118 = Unbundle By Name(w140) -> ("Yaw"=w128:dbl)
        "Yaw" <- w128
        n119 = call <vilib>:"Displacement.vi"("NavX Info In"=w135) -> ("Displacement"=→"Displacement":T1, "NavX Info Out"=w133:T25)  [unwired: 9 in]
        n120 = call "New motor Control integrated remodeled state based with PID.vi"("Yaw"=w128, "States"=w129) -> ("Speed and distance cluster"=w127:T2)  [unwired: 1 in, 1 out]
        "Speed and distance cluster" <- w127
        n121 = case shown="True" w157 {
          tunnel: w165 -> [w172 w184]
          tunnel: w148 -> [w173 w183]
          tunnel: w154 -> [w171 w179]
          tunnel: [w173 w183] -> w161
          tunnel: [w171 w194] -> w160
          tunnel: [w172 w193] -> w159
          tunnel: w155 -> [_ w192]
          tunnel: w158 -> [_ w191]
          tunnel: w151 -> [w170 w186]
          tunnel: [w170 w186] -> w150
          tunnel: [enum16{"OFF", "ON", "BLINK"}."BLINK" ("GREEN LED State") w180] -> w145
          tunnel: w127 -> [_ w177]
          tunnel: [_ w175] -> w144
          tunnel: w128 -> [_ w174]
          frame False {
          }
          frame True {
            # ">>State Logic Queue Reference >>"
            n122 = Get Queue Status(queue=w183) -> (error out=w182:errorcluster)  [unwired: 2 in, 7 out]
            n123 = local read "DIO 1"() -> (w181:bool)
            n124 = Unbundle(w177) -> (w176:T28)  [unwired: 1 out]
            n125 = case shown="No Error" w182 {
              tunnel: [w195 TLB_MHL_States."Reset" ("Enum")] -> w185
              tunnel: w184 -> [w195 _]
              frame No Error {
              }
              frame Error {
              }
            }
            n126 = Unbundle By Name(w186) -> ("Front Ultrasonic Obstruct"=w187:bool, "Right Ultrasonic Obstruct"=w178:bool)  [unwired: 1 out]
            n127 = Unbundle By Name(w176) -> ("xDistance"=w188:dbl, "yDistance"=w190:dbl, "wDistance"=w189:dbl)
            n128 = case shown="\"Autodrive\"" w185 {
              tunnel: w183 -> [w200 w265 w276 w293 w312 w328 w343 w359 w375 w391 _ w415 w437 w450 _ _ _ _]
              tunnel: w179 -> [_ w268 w282 w297 w321 w332 w348 w365 w380 w397 w408 w418 w438 w454 w463 w467 w473 w487]
              tunnel: [w197 w267 w281 w298 w320 w333 w347 w364 w379 w396 w407 w419 w439 w453 w463 w466 w473 w488] -> w194
              tunnel: [w203 TLB_MHL_States."Idle" ("Enum") w284 w299 w317 w336 w350 w363 w381 w395 TLB_MHL_States."Shutdown" ("Enum") w421 w430 w452 TLB_MHL_States."Reset" ("Enum") TLB_MHL_States."Shutdown" ("Enum") TLB_MHL_States."Reset" ("Enum") w484] -> w193
              tunnel: w192 -> [w201 _ _ _ _ _ _ _ _ _ _ _ _ _ _ _ _ _]
              tunnel: w191 -> [w202 _ _ _ _ _ _ _ _ _ _ _ _ _ _ _ _ _]
              tunnel: w181 -> [_ _ w279 w296 w315 _ _ _ _ w394 _ w416 w433 w451 _ _ _ w476]
              tunnel: w190 -> [_ _ w274 _ _ _ w342 w358 _ _ _ _ _ _ _ _ _ _]
              tunnel: w189 -> [_ _ _ _ w310 _ _ _ _ _ _ _ _ _ _ _ _ _]
              tunnel: w188 -> [_ _ _ _ _ _ _ _ w374 _ _ _ _ _ _ _ _ _]
              tunnel: w187 -> [_ _ _ w294 _ w330 _ _ _ w393 _ _ w432 _ _ _ _ _]
              tunnel: [enum16{"OFF", "ON", "BLINK"}."ON" ("GREEN LED State") enum16{"OFF", "ON", "BLINK"}."OFF" ("GREEN LED State") enum16{"OFF", "ON", "BLINK"}."BLINK" ("GREEN LED State") enum16{"OFF", "ON", "BLINK"}."BLINK" ("GREEN LED State") enum16{"OFF", "ON", "BLINK"}."BLINK" ("GREEN LED State") enum16{"OFF", "ON", "BLINK"}."BLINK" ("GREEN LED State") enum16{"OFF", "ON", "BLINK"}."BLINK" ("GREEN LED State") enum16{"OFF", "ON", "BLINK"}."BLINK" ("GREEN LED State") enum16{"OFF", "ON", "BLINK"}."BLINK" ("GREEN LED State") enum16{"OFF", "ON", "BLINK"}."BLINK" ("GREEN LED State") enum16{"OFF", "ON", "BLINK"}."OFF" ("GREEN LED State") enum16{"OFF", "ON", "BLINK"}."BLINK" ("GREEN LED State") enum16{"OFF", "ON", "BLINK"}."BLINK" ("GREEN LED State") enum16{"OFF", "ON", "BLINK"}."BLINK" ("GREEN LED State") _ enum16{"OFF", "ON", "BLINK"}."OFF" ("GREEN LED State") _ _] -> w180
              tunnel: w179 -> [w198 _ _ _ _ _ _ _ _ _ _ _ _ _ _ _ _ _]
              tunnel: w178 -> [_ _ _ _ _ _ _ _ _ _ _ _ _ _ _ _ _ _]
              tunnel: [_ _ _ _ _ _ _ _ _ _ _ _ w428 _ _ _ _ _] -> w175
              tunnel: w174 -> [_ _ _ _ _ _ _ _ _ _ _ _ _ _ _ _ _ w475]
              frame "Idle", Default {
                # ">>State Logic >>"
                n129 = Dequeue Element(queue=w200, timeout in ms (-1)=w202, error in (no error)=w201) -> (element=w204:T4)  [unwired: 3 out]
                "element" <- w204
                n130 = case shown="\"Start Drive Straight\"" w204 {
                  tunnel: [TLB_MHL_States."Idle" ("Enum") TLB_MHL_States."Idle" ("Enum") TLB_MHL_States."Task 1" ("Enum") TLB_MHL_States."Task 2" ("Enum") TLB_MHL_States."Task 3" ("Enum") TLB_MHL_States."Task 4" ("Enum") TLB_MHL_States."Shutdown" ("Enum") TLB_MHL_States."Wall follow mode" ("Enum") TLB_MHL_States."Acquire image" ("Enum") TLB_MHL_States."Autodrive" ("Enum")] -> w203
                  tunnel: w198 -> [w205 w207 w211 w218 w224 w232 w239 w246 w253 w260]
                  tunnel: [w205 w207 w210 w217 w225 w231 w238 w245 w252 w258] -> w197
                  frame "Start Sequence" {
                    # "This event should never be triggered"
                  }
                  frame "Idle", Default {
                    # ">>Action states Queue Reference >>"
                  }
                  frame "Start Task 1" {
                    # ">>Action states Queue Reference >>"
                    # "Action items"
                    n131 = for {
                      shift-right: [w215] -> w210
                      shift-left: w211 -> [w214]
                      tunnel: string[] ["Hardware reset", "Software reset", "Forward", ""] -> [w213] mode=indexing
                      n132 = Enqueue Element(queue=w214, element=w213) -> (queue out=w215:refnum<queue>)  [unwired: 2 in, 2 out]
                    }
                  }
                  frame "Start Task 2" {
                    # ">>Action states Queue Reference >>"
                    # "Action items"
                    n133 = for {
                      shift-right: [w222] -> w217
                      shift-left: w218 -> [w221]
                      tunnel: string[] ["Hardware reset", "Software reset", ""] -> [w220] mode=indexing
                      n134 = Enqueue Element(queue=w221, element=w220) -> (queue out=w222:refnum<queue>)  [unwired: 2 in, 2 out]
                    }
                  }
                  frame "Start Task 3" {
                    # ">>Action states Queue Reference >>"
                    n135 = for {
                      shift-right: [w229] -> w225
                      shift-left: w224 -> [w228]
                      tunnel: string[] ["Hardware reset", "Software reset", ""] -> [w227] mode=indexing
                      n136 = Enqueue Element(queue=w228, element=w227) -> (queue out=w229:refnum<queue>)  [unwired: 2 in, 2 out]
                    }
                  }
                  frame "Start Task 4" {
                    # ">>Action states Queue Reference >>"
                    # "Action items"
                    n137 = for {
                      shift-right: [w236] -> w231
                      shift-left: w232 -> [w235]
                      tunnel: string[] ["Hardware reset", "Software reset", ""] -> [w234] mode=indexing
                      n138 = Enqueue Element(queue=w235, element=w234) -> (queue out=w236:refnum<queue>)  [unwired: 2 in, 2 out]
                    }
                  }
                  frame "Exit" {
                    # ">>Action states Queue Reference >>"
                    # "Action items"
                    n139 = for {
                      shift-right: [w243] -> w238
                      shift-left: w239 -> [w242]
                      tunnel: string[] ["Hardware reset", "Software reset", "Motor Control", "Pre-Exit", "Exit"] -> [w241] mode=indexing
                      n140 = Enqueue Element(queue=w242, element=w241) -> (queue out=w243:refnum<queue>)  [unwired: 2 in, 2 out]
                    }
                  }
                  frame "Wall follow mode" {
                    # ">>Action states Queue Reference >>"
                    # "Action items"
                    n141 = for {
                      shift-right: [w250] -> w245
                      shift-left: w246 -> [w249]
                      tunnel: string[] ["Hardware reset", "Software reset", ""] -> [w248] mode=indexing
                      n142 = Enqueue Element(queue=w249, element=w248) -> (queue out=w250:refnum<queue>)  [unwired: 2 in, 2 out]
                    }
                  }
                  frame "Camera vision" {
                    # ">>Action states Queue Reference >>"
                    # "Action items"
                    n143 = for {
                      shift-right: [w257] -> w252
                      shift-left: w253 -> [w256]
                      tunnel: string[] ["Hardware reset", "Software reset", "Cam Init", "Cam Acq"] -> [w255] mode=indexing
                      n144 = Enqueue Element(queue=w256, element=w255) -> (queue out=w257:refnum<queue>)  [unwired: 2 in, 2 out]
                    }
                  }
                  frame "Start Drive Straight" {
                    # ">>Action states Queue Reference >>"
                    # "Action items"
                    n145 = for {
                      shift-right: [w264] -> w258
                      shift-left: w260 -> [w263]
                      tunnel: string[] ["Hardware reset", "Software reset", "Forward", ""] -> [w262] mode=indexing
                      n146 = Enqueue Element(queue=w263, element=w262) -> (queue out=w264:refnum<queue>)  [unwired: 2 in, 2 out]
                    }
                  }
                }
              }
              frame "Startup" {
                # ">>State Logic >>"
                n147 = Flush Queue(queue=w265) -> ()  [unwired: 1 in, 3 out]
                n148 = for {
                  shift-right: [w272] -> w267
                  shift-left: w268 -> [w273]
                  tunnel: string[] ["Init", "NavX Calibrate", "Software reset", "Hardware reset", "Motor Control"] -> [w271] mode=indexing
                  n149 = Enqueue Element(queue=w273, element=w271) -> (queue out=w272:refnum<queue>)  [unwired: 2 in, 2 out]
                }
              }
              frame "Task 1" {
                # ">>State Logic >>"
                n150 = Greater Or Equal?(x=w274, y=1.0) -> (x >= y?=w277:bool)
                n151 = Or(x=w279, y=w277) -> (x .or. y?=w280:bool)
                n152 = case shown="True" w280 {
                  tunnel: [string[] ["Forward", "Motor Control", ""] string[] ["Software reset", "Hardware reset", "Motor Control"]] -> w283
                  frame False {
                  }
                  frame True {
                  }
                }
                n153 = Flush Queue(queue=w276) -> ()  [unwired: 1 in, 3 out]
                n154 = Select(t=TLB_MHL_States."Idle" ("Enum"), s=w280, f=TLB_MHL_States."Task 1" ("Enum")) -> (s? t:f=w284:T5)
                n155 = for {
                  shift-right: [w290] -> w281
                  shift-left: w282 -> [w291]
                  tunnel: w283 -> [w289] mode=indexing
                  n156 = Enqueue Element(queue=w291, element=w289) -> (queue out=w290:refnum<queue>)  [unwired: 2 in, 2 out]
                }
              }
              frame "Task 2" {
                # ">>State Logic >>"
                n157 = Flush Queue(queue=w293) -> ()  [unwired: 1 in, 3 out]
                n158 = case shown="True" w296 {
                  tunnel: [w303 string[] ["Hardware reset", "Software reset", "Motor control"]] -> w295
                  tunnel: w294 -> [w302 _]
                  frame False {
                    n159 = case shown="False" w302 {
                      tunnel: [string[] ["Stop", "Ultrasonic read", "Motor Control"] string[] ["Reverse", "Ultrasonic read", "Motor control"]] -> w303
                      frame False {
                      }
                      frame True {
                      }
                    }
                  }
                  frame True {
                  }
                }
                n160 = Select(t=TLB_MHL_States."Idle" ("Enum"), s=w296, f=TLB_MHL_States."Task 2" ("Enum")) -> (s? t:f=w299:T5)
                n161 = for {
                  shift-right: [w308] -> w298
                  shift-left: w297 -> [w309]
                  tunnel: w295 -> [w307] mode=indexing
                  n162 = Enqueue Element(queue=w309, element=w307) -> (queue out=w308:refnum<queue>)  [unwired: 2 in, 2 out]
                }
              }
              frame "Task 3" {
                n163 = Greater Or Equal?(x=w310, y=360.0) -> (x >= y?=w314:bool)
                n164 = Flush Queue(queue=w312) -> ()  [unwired: 1 in, 3 out]
                n165 = Or(x=w314, y=w315) -> (x .or. y?=w316:bool)
                n166 = case shown="False" w316 {
                  tunnel: [string[] ["Rotate CW", "Motor Control"] string[] ["Software reset", "Hardware reset", "Motor Control"]] -> w322
                  frame False {
                  }
                  frame True {
                  }
                }
                n167 = for {
                  shift-right: [w324] -> w320
                  shift-left: w321 -> [w325]
                  tunnel: w322 -> [w323] mode=indexing
                  n168 = Enqueue Element(queue=w325, element=w323) -> (queue out=w324:refnum<queue>)  [unwired: 2 in, 2 out]
                }
                n169 = Select(t=TLB_MHL_States."Idle" ("Enum"), s=w316, f=TLB_MHL_States."Task 3" ("Enum")) -> (s? t:f=w317:T5)
              }
              frame "Task 4" {
                n170 = Flush Queue(queue=w328) -> ()  [unwired: 1 in, 3 out]
                n171 = case shown="True" w330 {
                  tunnel: [string[] ["Forward", "Ultrasonic read", "Motor Control"] string[] ["Stop", "Hardware reset", "Software reset", "Motor Control"]] -> w331
                  frame False {
                  }
                  frame True {
                  }
                }
                n172 = for {
                  shift-right: [w340] -> w333
                  shift-left: w332 -> [w341]
                  tunnel: w331 -> [w339] mode=indexing
                  n173 = Enqueue Element(queue=w341, element=w339) -> (queue out=w340:refnum<queue>)  [unwired: 2 in, 2 out]
                }
                n174 = Select(t=TLB_MHL_States."Task 4a" ("Enum"), s=w330, f=TLB_MHL_States."Task 4" ("Enum")) -> (s? t:f=w336:T5)
              }
              frame "Task 4a" {
                n175 = Greater Or Equal?(x=w342, y=0.5) -> (x >= y?=w346:bool)
                n176 = Flush Queue(queue=w343) -> ()  [unwired: 1 in, 3 out]
                n177 = case shown="True" w346 {
                  tunnel: [string[] ["Right", "Motor Control"] string[] ["Stop", "Hardware reset", "Software reset", "Motor Control"]] -> w349
                  frame False {
                  }
                  frame True {
                  }
                }
                n178 = for {
                  shift-right: [w356] -> w347
                  shift-left: w348 -> [w357]
                  tunnel: w349 -> [w355] mode=indexing
                  n179 = Enqueue Element(queue=w357, element=w355) -> (queue out=w356:refnum<queue>)  [unwired: 2 in, 2 out]
                }
                n180 = Select(t=TLB_MHL_States."Task 4b" ("Enum"), s=w346, f=TLB_MHL_States."Task 4a" ("Enum")) -> (s? t:f=w350:T5)
              }
              frame "Task 4b" {
                n181 = Flush Queue(queue=w359) -> ()  [unwired: 1 in, 3 out]
                n182 = Greater Or Equal?(x=w358, y=0.75) -> (x >= y?=w361:bool)
                n183 = case shown="False" w361 {
                  tunnel: [string[] ["Forward", "Motor control"] string[] ["Stop", "Hardware reset", "Software reset"]] -> w366
                  frame False {
                  }
                  frame True {
                  }
                }
                n184 = for {
                  shift-right: [w372] -> w364
                  shift-left: w365 -> [w373]
                  tunnel: w366 -> [w371] mode=indexing
                  n185 = Enqueue Element(queue=w373, element=w371) -> (queue out=w372:refnum<queue>)  [unwired: 2 in, 2 out]
                }
                n186 = Select(t=TLB_MHL_States."Task 4c" ("Enum"), s=w361, f=TLB_MHL_States."Task 4b" ("Enum")) -> (s? t:f=w363:T5)
              }
              frame "Task 4c" {
                n187 = Flush Queue(queue=w375) -> ()  [unwired: 1 in, 3 out]
                n188 = Less Or Equal?(x=w374, y=-0.65) -> (x <= y?=w377:bool)
                n189 = case shown="False" w377 {
                  tunnel: [string[] ["Left", "Motor Control"] string[] ["Stop", "Hardware reset", "Software reset", "Motor Control"]] -> w382
                  frame False {
                  }
                  frame True {
                  }
                }
                n190 = for {
                  shift-right: [w388] -> w379
                  shift-left: w380 -> [w389]
                  tunnel: w382 -> [w387] mode=indexing
                  n191 = Enqueue Element(queue=w389, element=w387) -> (queue out=w388:refnum<queue>)  [unwired: 2 in, 2 out]
                }
                n192 = Select(t=TLB_MHL_States."Task 4d" ("Enum"), s=w377, f=TLB_MHL_States."Task 4c" ("Enum")) -> (s? t:f=w381:T5)
              }
              frame "Task 4d" {
                n193 = Flush Queue(queue=w391) -> ()  [unwired: 1 in, 3 out]
                n194 = Or(x=w394, y=w393) -> (x .or. y?=w392:bool)
                n195 = case shown="True" w392 {
                  tunnel: [string[] ["Forward", "Ultrasonic Read", "Motor Control"] string[] ["Stop", "Hardware reset", "Software reset", "Motor Control"]] -> w398
                  frame False {
                  }
                  frame True {
                  }
                }
                n196 = for {
                  shift-right: [w404] -> w396
                  shift-left: w397 -> [w405]
                  tunnel: w398 -> [w403] mode=indexing
                  n197 = Enqueue Element(queue=w405, element=w403) -> (queue out=w404:refnum<queue>)  [unwired: 2 in, 2 out]
                }
                n198 = Select(t=TLB_MHL_States."Idle" ("Enum"), s=w392, f=TLB_MHL_States."Task 4d" ("Enum")) -> (s? t:f=w395:T5)
              }
              frame "Reset" {
                n199 = for {
                  shift-right: [w412] -> w407
                  shift-left: w408 -> [w413]
                  tunnel: string[] ["Software reset", "Hardware reset", "Motor Control"] -> [w411] mode=indexing
                  n200 = Enqueue Element(queue=w413, element=w411) -> (queue out=w412:refnum<queue>)  [unwired: 2 in, 2 out]
                }
              }
              frame "Wall follow mode" {
                n201 = Flush Queue(queue=w415) -> ()  [unwired: 1 in, 3 out]
                n202 = case shown="False" w416 {
                  tunnel: [string[] ["IR Sensor Read", "Calculate", "Forward", "Motor Control"] string[] ["Hardware reset", "Software reset", "Motor Control"]] -> w417
                  frame False {
                  }
                  frame True {
                  }
                }
                n203 = for {
                  shift-right: [w426] -> w419
                  shift-left: w418 -> [w427]
                  tunnel: w417 -> [w425] mode=indexing
                  n204 = Enqueue Element(queue=w427, element=w425) -> (queue out=w426:refnum<queue>)  [unwired: 2 in, 2 out]
                }
                n205 = Select(t=TLB_MHL_States."Idle" ("Enum"), s=w416, f=TLB_MHL_States."Wall follow mode" ("Enum")) -> (s? t:f=w421:T5)
              }
              frame "Autodrive" {
                # ">>>Return to idle event>>>"
                n206 = Flush Queue(queue=w437) -> ()  [unwired: 1 in, 3 out]
                n207 = Boolean To (0,1)(Boolean=w433) -> (0, 1=w435:i16)
                n208 = Boolean To (0,1)(Boolean=w432) -> (0, 1=w434:i16)
                n209 = formula code="int8  out;\nif (detect == 0 && stop == 0)\nout = 0;\n\nelse if (detect == 1 && stop == 0)\nout = 1;\n\nelse if (detect == 0 && stop == 1)\nout = 2;\n\nelse\nout = 0;"("stop"=w435, "detect"=w434) -> ("out"=w428:i8)
                n210 = case shown="2" w428 {
                  tunnel: [string[] ["Forward", "Ultrasonic read"] string[] ["Hardware reset", "Software reset", "Rotate Clockwise", ""] string[] ["Stop", "", "Software reset", "Motor Control"]] -> w431
                  frame 0, Default {
                  }
                  frame 1 {
                  }
                  frame 2 {
                  }
                }
                n211 = call "Servo State FGV.vi"("Init/Read/Write State"=States_for_Action_Engine."Write", "Servo State"=w428) -> ()  [unwired: 1 in, 2 out]
                n212 = for {
                  shift-right: [w447] -> w439
                  shift-left: w438 -> [w448]
                  tunnel: w431 -> [w446] mode=indexing
                  n213 = Enqueue Element(queue=w448, element=w446) -> (queue out=w447:refnum<queue>)  [unwired: 2 in, 2 out]
                }
                n214 = case shown="2" w428 {
                  tunnel: [TLB_MHL_States."Autodrive" ("Enum") TLB_MHL_States."Autodrive a" ("Enum") TLB_MHL_States."Idle" ("Enum")] -> w430
                  frame 0, Default {
                  }
                  frame 1 {
                  }
                  frame 2 {
                  }
                }
              }
              frame "Acquire image" {
                n215 = Flush Queue(queue=w450) -> ()  [unwired: 1 in, 3 out]
                n216 = case shown="True" w451 {
                  tunnel: [string[] ["Cam Acq"] string[] ["Hardware reset", "Software reset", "Cam Exit", ""]] -> w455
                  frame False {
                  }
                  frame True {
                  }
                }
                n217 = for {
                  shift-right: [w461] -> w453
                  shift-left: w454 -> [w462]
                  tunnel: w455 -> [w460] mode=indexing
                  n218 = Enqueue Element(queue=w462, element=w460) -> (queue out=w461:refnum<queue>)  [unwired: 2 in, 2 out]
                }
                n219 = Select(t=TLB_MHL_States."Idle" ("Enum"), s=w451, f=TLB_MHL_States."Acquire image" ("Enum")) -> (s? t:f=w452:T5)
              }
              frame "Processing" {
              }
              frame "Shutdown" {
                # ">>State Logic >>"
                n220 = for {
                  shift-right: [w471] -> w466
                  shift-left: w467 -> [w472]
                  tunnel: string[] ["Software reset", "Hardware reset", "Motor Control", "Cam Exit", "Pre-Exit", "Exit"] -> [w470] mode=indexing
                  n221 = Enqueue Element(queue=w472, element=w470) -> (queue out=w471:refnum<queue>)  [unwired: 2 in, 2 out]
                }
              }
              frame "None" {
              }
              frame "Autodrive a" {
                n222 = Greater Or Equal?(x=w475, y=80.0) -> (x >= y?=w477:bool)
                n223 = Or(x=w476, y=w477) -> (x .or. y?=w478:bool)
                n224 = case shown="True" w478 {
                  tunnel: [string[] ["Rotate CW", "Ultrasonic read", ""] string[] ["Stop", "", "Software reset", ""]] -> w486
                  frame False {
                  }
                  frame True {
                  }
                }
                n225 = for {
                  shift-right: [w492] -> w488
                  shift-left: w487 -> [w493]
                  tunnel: w486 -> [w491] mode=indexing
                  n226 = Enqueue Element(queue=w493, element=w491) -> (queue out=w492:refnum<queue>)  [unwired: 2 in, 2 out]
                }
                n227 = Or(x=w476, y=w477) -> (x .or. y?=w479:bool)
                n228 = Select(t=TLB_MHL_States."Idle" ("Enum"), s=w476, f=TLB_MHL_States."Autodrive" ("Enum")) -> (s? t:f=w482:T5)
                n229 = Select(t=w482, s=w479, f=TLB_MHL_States."Autodrive a" ("Enum")) -> (s? t:f=w484:T5)
              }
            }
          }
        }
        n230 = call "Servo State FGV.vi"("Init/Read/Write State"=States_for_Action_Engine."Read") -> ("Output"=→"Output":dbl)  [unwired: 2 in, 1 out]
        n231 = local write "GREEN LED State"(w145) -> ()
        "Decision" <- w143
      }
      n232 = while {
        shift-right: [w110] -> _
        shift-left: _ -> [w111]
        shift-right: [w109] -> _
        shift-left: _ -> [w108]
        stop <- w117 stop-if-true
        (unwired) TRUE
        # "LED Blinker Loop"
        n233 = case shown="\"BLINK\"" "GREEN LED State" {
          tunnel: [FALSE TRUE w125] -> w113
          tunnel: w111 -> [_ _ w125]
          tunnel: [_ _ w126] -> w110
          frame "OFF", Default {
          }
          frame "ON" {
          }
          frame "BLINK" {
            n234 = Not(x=w125) -> (.not. x?=w126:bool)
          }
        }
        n235 = case shown="\"OFF\", Default" "RED LED State" {
          tunnel: [FALSE TRUE w121] -> w112
          tunnel: [_ _ w122] -> w109
          tunnel: w108 -> [_ _ w121]
          frame "OFF", Default {
          }
          frame "ON" {
          }
          frame "BLINK" {
            n236 = Not(x=w121) -> (.not. x?=w122:bool)
          }
        }
        n237 = local write "Green LED"(w113) -> ()
        n238 = local write "Red LED"(w112) -> ()
        n239 = call "FGV Bool.vi"("Init/Read/Write State"=States_for_Action_Engine."Read") -> ("Output node"=w117:bool)  [unwired: 2 in, 1 out]
        n240 = Wait (ms)(milliseconds to wait=u32 500) -> ()  [unwired: 1 out]
      }
      n241 = call <vilib>:"DIO Close.vi"("DIO Info In"=w6) -> ()  [unwired: 10 in, 1 out]
      n242 = call <vilib>:"DIO Close.vi"("error in (no error)"=w23, "DIO Info In"=w29) -> ()  [unwired: 9 in, 1 out]
      n243 = call <vilib>:"DIO Close.vi"("error in (no error)"=w21, "DIO Info In"=w25) -> ()  [unwired: 9 in, 1 out]
      n244 = call <vilib>:"DIO Close.vi"("error in (no error)"=w11, "DIO Info In"=w16) -> ()  [unwired: 9 in, 1 out]
      n245 = call <vilib>:"DIO Close.vi"("error in (no error)"=w9, "DIO Info In"=w15) -> ()  [unwired: 9 in, 1 out]
      n246 = disable-structure shown="Disabled" {
        frame Disabled {
          n247 = call <vilib>:"FPGA Open.vi"() -> ("error out"=w65:errorcluster, "FPGA Reference Out"=w64:refnum<k20>)  [unwired: 10 in]
          n248 = call <vilib>:"I2C Config.vi"("error in (no error)"=w65, "FPGA Reference"=w64) -> ("error out"=w62:errorcluster, "I2C Ref Out"=w63:T22)  [unwired: 8 in]
          n249 = while {
            tunnel: w63 -> [w67]
            tunnel: w62 -> [w66]
            stop <- _ stop-if-true
            n250 = call <vilib>:"I2C Write.vi"("error in (no error)"=w66, "I2C Ref In"=w67) -> ()  [unwired: 8 in, 2 out]
          }
        }
        frame Enabled {
        }
      }
      n251 = Merge Errors "Merge Errors"(w55, w54) -> (w36:errorcluster)
      n252 = Merge Errors(w40, w36) -> (w31:errorcluster)
      n253 = Destroy User Event(user event=w58, error in=w31) -> ()  [unwired: 1 out]
      n254 = Destroy User Event(user event=w59, error in=w31) -> ()  [unwired: 1 out]
      n255 = Unregister For Events(event registration refnum=w50, error in=w31) -> ()  [unwired: 1 out]
      n256 = Release Queue(queue=w33, error in (no error)=w31) -> (error out=→"error out":errorcluster)  [unwired: 1 in, 2 out]
      n257 = call <vilib>:"NavX Close.vi"("NavX Info In"=w5) -> ()  [unwired: 10 in, 1 out]
      n258 = Release Queue(queue=w49, error in (no error)=w31) -> ()  [unwired: 1 in, 3 out]
    }
    frame #2 {
      n259 = call "New motor Control integrated remodeled state based with PID.vi"("States"=States_for_motor_control."INIT") -> ()  [unwired: 2 in, 2 out]
    }
    frame #3 {
    }
  }
